vi "experienceInfo.vi"(10 "info in":string, 11 "Experiments":T1(array[cluster])) -> (3 "info out":string)   [LabVIEW 2019]
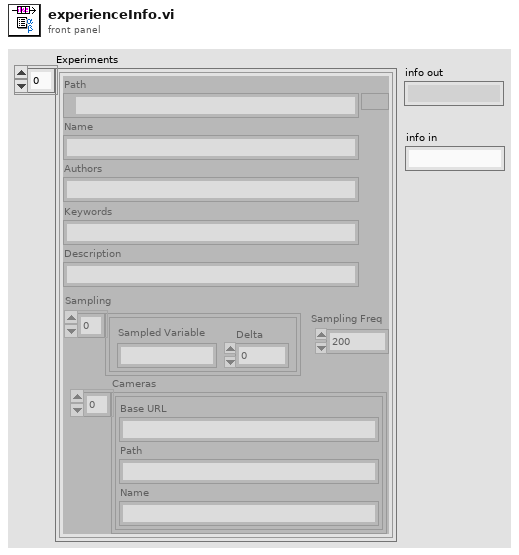
[diagram p1: front panel]
types:
  T1 = cluster{"Path":path, "Name":string, "Authors":string, "Keywords":string, "Description":string, "Cameras":cluster{"Base URL":string, "Path":string, "Name":string}[], "Sampling":cluster{"Sampled Variable":string, "Delta":dbl}[], "Sampling Freq":u32}[]
  T2 = cluster{"Name":string, "Type":string, "Min":string, "Max":string, "Precision":string, "Description":string}[]
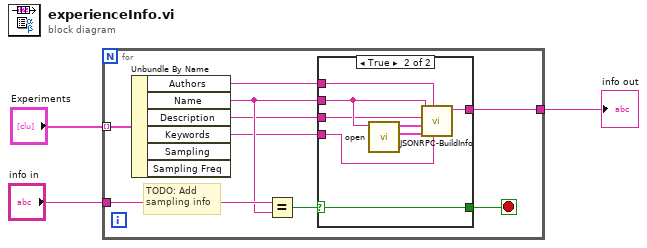
[diagram p0: block diagram]
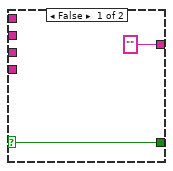
[diagram p2: hidden frame]
diagram:
  n1 = for {
    tunnel: "Experiments" -> [w12] mode=indexing
    tunnel: "info in" -> [w11]
    tunnel: [w4] -> w3
    stop <- w8 stop-if-true
    # "TODO: Add\nsampling info"
    n2 = Unbundle By Name(w12) -> ("Authors"=w7:string, "Name"=w10:string, "Description"=w6:string, "Keywords"=w5:string)  [unwired: 2 out]
    n3 = Equal?(x=w11, y=w10) -> (x = y?=w9:bool)
    n4 = case shown="True" w9 {
      selector: w9 -> [w13 w18]
      tunnel: w10 -> [_ w20]
      tunnel: w6 -> [_ w17]
      tunnel: w5 -> [_ w15]
      tunnel: w7 -> [_ w16]
      tunnel: ["" ("info") w19] -> w4
      tunnel: [w13 w18] -> w8
      frame False {
      }
      frame True {
        n5 = call "open.vi"("Experience ID"=w20) -> ("Indicators_list"=w22:T2, "Controls_list"=w21:T2)  [unwired: 8 in, 1 out]
        n6 = call "JSONRPC-BuildInfo.vi"("keywords"=w15, "authors"=w16, "readables"=w22, "writables"=w21, "description"=w17, "expId"=w20) -> ("info"=w19:string)  [unwired: 5 in]
      }
    }
  }
  "info out" <- w3
